vi "Valve_EPICS_Dev4_APX - Copy.vi"() -> ()   [LabVIEW 2015]
uses:
  <vilib>/Platform/TimedLoop/XDataNode/timing_clust.ctl
  <vilib>/Platform/TimedLoop/XDataNode/nitl_modes.ctl
  <vilib>/Platform/TimedLoop/XDataNode/wakeup.ctl
  <userlib>/caLab/Private/Get_PV-1D.vi
  <userlib>/caLab/Private/Put_DBL-1D_PV-1D.vi
  <vilib>/platform/TimedLoop/XDataNode/XDataNode.xnode
  <vilib>/Platform/TimedLoop/XDataNode/XDNodeRunTimeDep.lvlib
panel:
  out "Vacuum_REQ":bool
  out "Ambient_REQ":bool
  out "V7_CLOSE_REQ":bool
  out "V6_CLOSE_REQ":bool
  out "V5_CLOSE_REQ":bool
  out "V4_CLOSE_REQ":bool
  out "V3_CLOSE_REQ":bool
  out "V2_CLOSE_REQ":bool
  out "V1_CLOSE_REQ":bool
  out "V0_CLOSE_REQ":bool
  out "V7_OPEN_REQ":bool
  out "V6_OPEN_REQ":bool
  out "V5_OPEN_REQ":bool
  out "V4_OPEN_REQ":bool
  out "V3_OPEN_REQ":bool
  out "V2_OPEN_REQ":bool
  out "V1_OPEN_REQ":bool
  out "V0_OPEN_REQ":bool
  out "V7_OPEN_ENB":bool
  out "V6_OPEN_ENB":bool
  out "V5_OPEN_ENB":bool
  out "V4_OPEN_ENB":bool
  out "V3_OPEN_ENB":bool
  out "V2_OPEN_ENB":bool
  out "V1_OPEN_ENB":bool
  out "V0_OPEN_ENB":bool
  out "Boolean array":bool[](array[boolean])
  out "V7_OPEN_ACT":bool
  out "V6_OPEN_ACT":bool
  out "V5_OPEN_ACT":bool
  out "V4_OPEN_ACT":bool
  out "V3_OPEN_ACT":bool
  out "V2_OPEN_ACT":bool
  out "V1_OPEN_ACT":bool
  out "V0_OPEN_ACT":bool
  out "initialized array":i16[](array[numeric])
  in  "stop":bool
  out "sum":i16
  out "0, 1":i16[](array[numeric])
  out "SCL_data":u32[](array[numeric]) caption="SCL"
  out "SOP_data":u32[](array[numeric]) caption="SOP"
  out "SCL7":bool
  out "SCL6":bool
  out "SCL5":bool
  out "SCL4":bool
  out "SCL3":bool
  out "SCL2":bool
  out "SCL1":bool
  out "SCL0":bool
  out "SOP7":bool
  out "SOP6":bool
  out "SOP5":bool
  out "SOP4":bool
  out "SOP3":bool
  out "SOP2":bool
  out "SOP1":bool
  out "SOP0":bool
  # "Valve control DEV4"
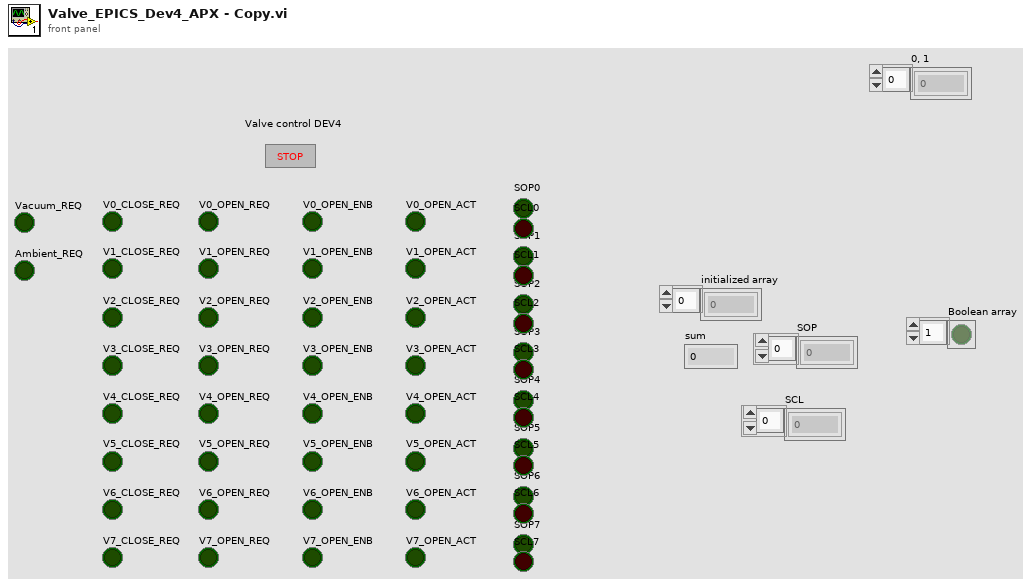
[diagram p1: front panel]
types:
  T1 = typedef "XDNodeRunTimeDep.lvlib/timing_clust.ctl" = cluster{"Expected End [f-1]":u64, "Actual End [f-1]":u64, "Finished Late? [f-1]":bool, "Expected End [i-1]":u64, "Actual End [i-1]":u64, "Finished Late? [i-1]":bool, "Expected Start [i]":u64, "Actual Start [i]":u64, "Expected Start [f]":u64, "Actual Start [f]":u64, "Source Name":string, "Structure Name":string, "Period":i64, "Deadline":i64, "Offset":i64, "Start":i64, "Priority":i32, "Timeout":i32, "Mode":T2, "Wakeup Reason":T3, "Error":errorcluster, "Source Type":string, "Secondary Source Type":string, "Global End Time":u64, "Global Start Time":u64, "Frame Duration":u64, "Iteration Duration":u64, "Assigned CPU":i32, "I/O Scan Engine Mode":u32}
  T2 = typedef "XDNodeRunTimeDep.lvlib/nitl_modes.ctl" = enum32{"No Change", "Process missed periods, maintain original phase", "Discard missed periods, maintain original phase", "Process missed periods, ignore original phase", "Discard missed periods, ignore original phase"}
  T3 = typedef "XDNodeRunTimeDep.lvlib/wakeup.ctl" = enum32{"Normal", "Aborted", "Asynchronous wakeup", "Timing source error", "Timed loop error", "Timeout"}
  T4 = typedef "NI_Matrix.lvlib/RealMatrix.ctl" = dbl[][]
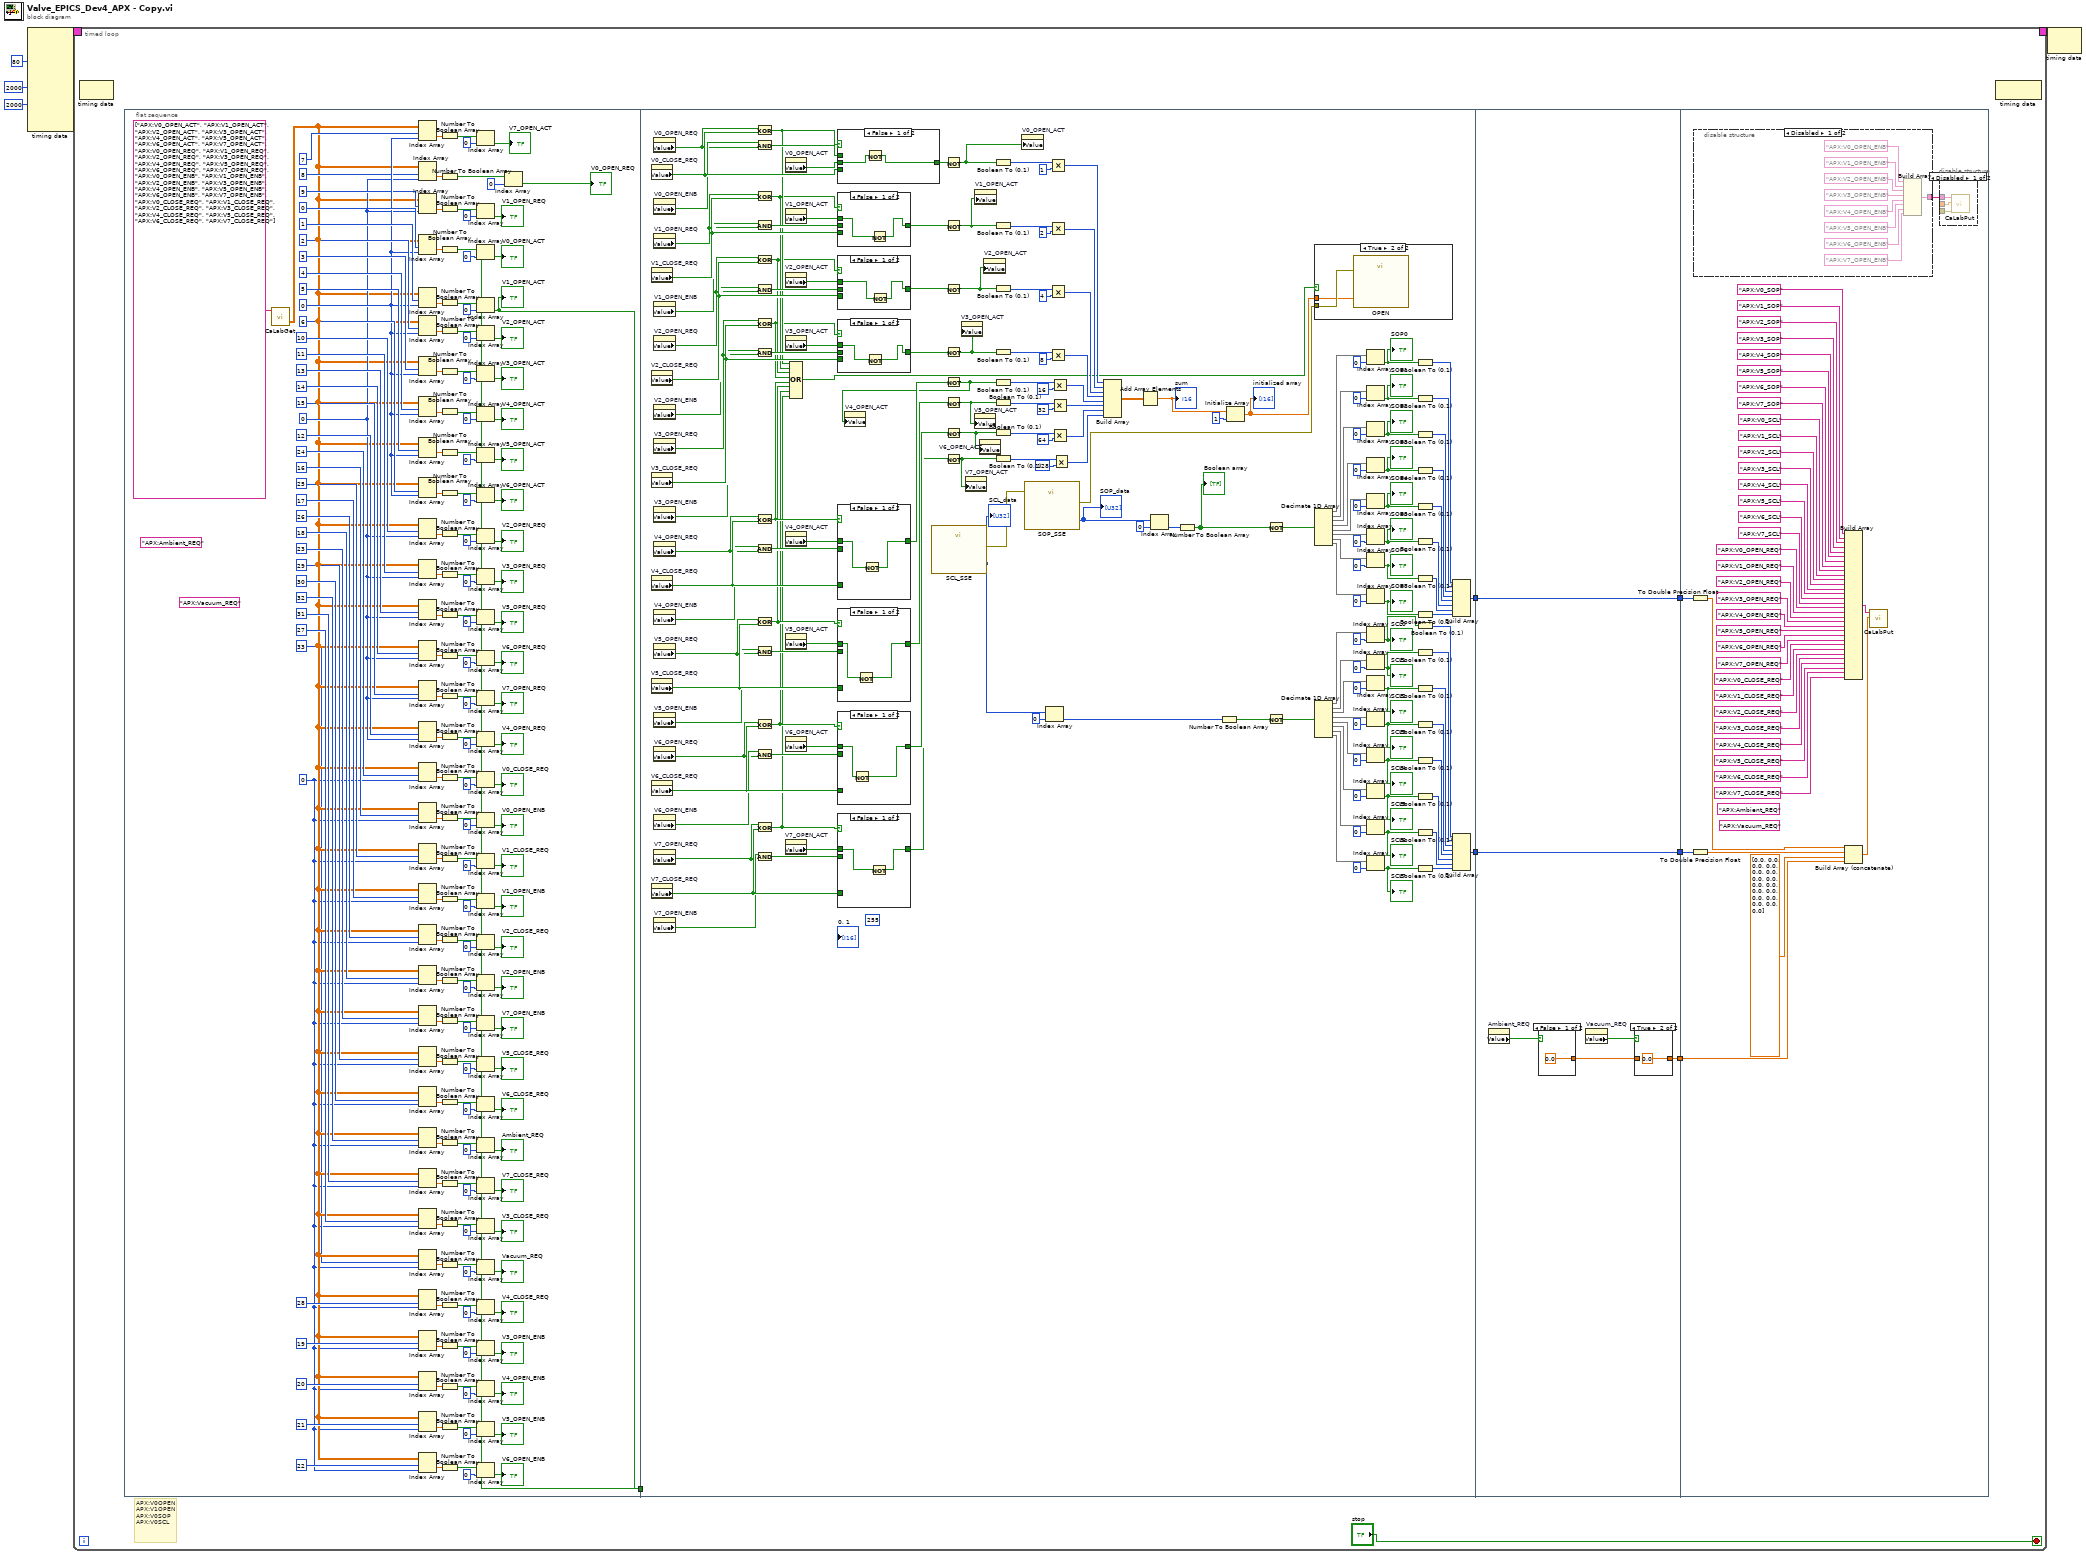
[diagram p0: block diagram]
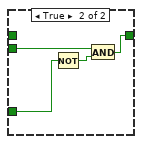
[diagram p3: hidden frame]
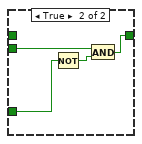
[diagram p4: hidden frame]
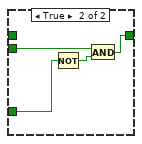
[diagram p5: hidden frame]
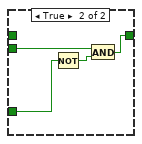
[diagram p6: hidden frame]
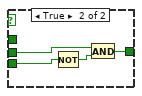
[diagram p7: hidden frame]
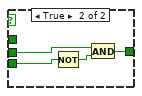
[diagram p8: hidden frame]
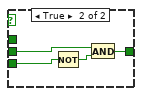
[diagram p9: hidden frame]
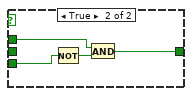
[diagram p10: hidden frame]
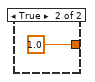
[diagram p12: hidden frame]
diagram:
  n1 = node-c288(80 ("Priority"), i64 2000 ("Deadline"), 2000 ("Timeout")) -> (w5:T1)  [unwired: 7 in]
  n2 = timed-loop {
    timing: w5 -> [_]
    timing-out: [_] -> w4
    stop <- "stop" stop-if-true
    # "APX:V0OPEN\nAPX:V1OPEN\nAPX:V0SOP\nAPX:V0SCL"
    n3 = node-c288() -> ()  [unwired: 1 in, 1 out]
    n4 = flat-sequence {
      tunnel: [w78] -> w18
      tunnel: [w77] -> w17
      tunnel: [w73] -> w16
      tunnel: [w80] -> w15
      tunnel: [w79] -> w14
      tunnel: [w76] -> w13
      tunnel: [w75] -> w12
      tunnel: w18 -> [_]
      tunnel: w17 -> [_]
      tunnel: w16 -> [_]
      tunnel: w15 -> [_]
      tunnel: w14 -> [_]
      tunnel: w13 -> [_]
      tunnel: w12 -> [_]
      tunnel: [w270] -> w11
      tunnel: [w343] -> w8
      tunnel: w11 -> [w422]
      tunnel: [w422] -> w10
      tunnel: w8 -> [w421]
      tunnel: [w421] -> w7
      tunnel: [w417] -> w6
      tunnel: w10 -> [w467]
      tunnel: w7 -> [w466]
      tunnel: w6 -> [w427]
      frame #0 {
        (unwired) "APX:Vacuum_REQ"
        (unwired) "APX:Ambient_REQ"
        w24 = 0 ("index")
        w153 = 0 ("index")
        w186 = 0 ("index")
        n5 = call-poly "CaLabGet.vi"("PV Names"=string[] ["APX:V0_OPEN_ACT", "APX:V1_OPEN_ACT", "APX:V2_OPEN_ACT", "APX:V3_OPEN_ACT", "APX:V4_OPEN_ACT", "APX:V5_OPEN_ACT", "APX:V6_OPEN_ACT", "APX:V7_OPEN_ACT", "APX:V0_OPEN_REQ", "APX:V1_OPEN_REQ", "APX:V2_OPEN_REQ", "APX:V3_OPEN_REQ", "APX:V4_OPEN_REQ", "APX:V5_OPEN_REQ", "APX:V6_OPEN_REQ", "APX:V7_OPEN_REQ", "APX:V0_OPEN_ENB", "APX:V1_OPEN_ENB", "APX:V2_OPEN_ENB", "APX:V3_OPEN_ENB", "APX:V4_OPEN_ENB", "APX:V5_OPEN_ENB", "APX:V6_OPEN_ENB", "APX:V7_OPEN_ENB", "APX:V0_CLOSE_REQ", "APX:V1_CLOSE_REQ", "APX:V2_CLOSE_REQ", "APX:V3_CLOSE_REQ", "APX:V4_CLOSE_REQ", "APX:V5_CLOSE_REQ", "APX:V6_CLOSE_REQ", "APX:V7_CLOSE_REQ"]) -> ("Value Array (number)"=w26:dbl[][])  [unwired: 8 in, 6 out]
        n6 = Index Array(array=w26, index (row)=7, index (col)=w186) -> (element=w162:dbl)
        n7 = Index Array(array=w26, index (row)=8 ("disabled index (row)"), index (col)=w153) -> (element=w133:dbl)
        n8 = Index Array(array=w26, index (row)=9, index (col)=w153) -> (element=w132:dbl)
        n9 = Index Array(array=w26, index (row)=0 ("disabled index (row)"), index (col)=w186) -> (element=w166:dbl)
        n10 = Index Array(array=w26, index (row)=1, index (col)=w186) -> (element=w165:dbl)
        n11 = Index Array(array=w26, index (row)=2, index (col)=w186) -> (element=w169:dbl)
        n12 = Index Array(array=w26, index (row)=3 ("index"), index (col)=w186) -> (element=w168:dbl)
        n13 = Index Array(array=w26, index (row)=4, index (col)=w186) -> (element=w167:dbl)
        n14 = Index Array(array=w26, index (row)=5, index (col)=w186) -> (element=w164:dbl)
        n15 = Index Array(array=w26, index (row)=6, index (col)=w186) -> (element=w163:dbl)
        n16 = Index Array(array=w26, index (row)=10, index (col)=w153) -> (element=w136:dbl)
        n17 = Index Array(array=w26, index (row)=11 ("index"), index (col)=w153) -> (element=w135:dbl)
        n18 = Index Array(array=w26, index (row)=13, index (col)=w153) -> (element=w131:dbl)
        n19 = Index Array(array=w26, index (row)=14, index (col)=w153) -> (element=w130:dbl)
        n20 = Index Array(array=w26, index (row)=15, index (col)=w153) -> (element=w129:dbl)
        n21 = Index Array(array=w26, index (row)=12, index (col)=w153) -> (element=w134:dbl)
        n22 = Index Array(array=w26, index (row)=24, index (col)=w24) -> (element=w53:dbl)
        n23 = Index Array(array=w26, index (row)=16 ("disabled index (row)"), index (col)=w24) -> (element=w101:dbl)
        n24 = Index Array(array=w26, index (row)=25, index (col)=w24) -> (element=w52:dbl)
        n25 = Index Array(array=w26, index (row)=17, index (col)=w24) -> (element=w100:dbl)
        n26 = Index Array(array=w26, index (row)=26, index (col)=w24) -> (element=w56:dbl)
        n27 = Index Array(array=w26, index (row)=18, index (col)=w24) -> (element=w104:dbl)
        n28 = Index Array(array=w26, index (row)=23, index (col)=w24) -> (element=w97:dbl)
        n29 = Index Array(array=w26, index (row)=29, index (col)=w24) -> (element=w51:dbl)
        n30 = Index Array(array=w26, index (row)=30, index (col)=w24) -> (element=w50:dbl)
        n31 = Index Array(array=w26, index (row)=32, index (col)=w24) -> (element=w30:dbl)
        n32 = Index Array(array=w26, index (row)=31, index (col)=w24) -> (element=w49:dbl)
        n33 = Index Array(array=w26, index (row)=27, index (col)=w24) -> (element=w55:dbl)
        n34 = Index Array(array=w26, index (row)=33, index (col)=w24) -> (element=w27:dbl)
        n35 = Index Array(array=w26, index (row)=28, index (col)=w24) -> (element=w54:dbl)
        n36 = Index Array(array=w26, index (row)=19 ("index"), index (col)=w24) -> (element=w103:dbl)
        n37 = Index Array(array=w26, index (row)=20, index (col)=w24) -> (element=w102:dbl)
        n38 = Index Array(array=w26, index (row)=21, index (col)=w24) -> (element=w99:dbl)
        n39 = Index Array(array=w26, index (row)=22, index (col)=w24) -> (element=w98:dbl)
        n40 = Number To Boolean Array(number=w162) -> (Boolean array=w171:bool[])
        n41 = Number To Boolean Array(number=w133) -> (Boolean array=w146:bool[])
        n42 = Number To Boolean Array(number=w132) -> (Boolean array=w144:bool[])
        n43 = Number To Boolean Array(number=w166) -> (Boolean array=w179:bool[])
        n44 = Number To Boolean Array(number=w165) -> (Boolean array=w177:bool[])
        n45 = Number To Boolean Array(number=w169) -> (Boolean array=w185:bool[])
        n46 = Number To Boolean Array(number=w168) -> (Boolean array=w183:bool[])
        n47 = Number To Boolean Array(number=w167) -> (Boolean array=w181:bool[])
        n48 = Number To Boolean Array(number=w164) -> (Boolean array=w175:bool[])
        n49 = Number To Boolean Array(number=w163) -> (Boolean array=w173:bool[])
        n50 = Number To Boolean Array(number=w136) -> (Boolean array=w152:bool[])
        n51 = Number To Boolean Array(number=w135) -> (Boolean array=w150:bool[])
        n52 = Number To Boolean Array(number=w131) -> (Boolean array=w142:bool[])
        n53 = Number To Boolean Array(number=w130) -> (Boolean array=w140:bool[])
        n54 = Number To Boolean Array(number=w129) -> (Boolean array=w138:bool[])
        n55 = Number To Boolean Array(number=w134) -> (Boolean array=w148:bool[])
        n56 = Number To Boolean Array(number=w53) -> (Boolean array=w66:bool[])
        n57 = Number To Boolean Array(number=w101) -> (Boolean array=w114:bool[])
        n58 = Number To Boolean Array(number=w52) -> (Boolean array=w64:bool[])
        n59 = Number To Boolean Array(number=w100) -> (Boolean array=w112:bool[])
        n60 = Number To Boolean Array(number=w56) -> (Boolean array=w72:bool[])
        n61 = Number To Boolean Array(number=w104) -> (Boolean array=w120:bool[])
        n62 = Number To Boolean Array(number=w97) -> (Boolean array=w106:bool[])
        n63 = Number To Boolean Array(number=w51) -> (Boolean array=w62:bool[])
        n64 = Number To Boolean Array(number=w50) -> (Boolean array=w60:bool[])
        n65 = Number To Boolean Array(number=w30) -> (Boolean array=w32:bool[])
        n66 = Number To Boolean Array(number=w49) -> (Boolean array=w58:bool[])
        n67 = Number To Boolean Array(number=w55) -> (Boolean array=w70:bool[])
        n68 = Number To Boolean Array(number=w27) -> (Boolean array=w23:bool[])
        n69 = Number To Boolean Array(number=w54) -> (Boolean array=w68:bool[])
        n70 = Number To Boolean Array(number=w103) -> (Boolean array=w118:bool[])
        n71 = Number To Boolean Array(number=w102) -> (Boolean array=w116:bool[])
        n72 = Number To Boolean Array(number=w99) -> (Boolean array=w110:bool[])
        n73 = Number To Boolean Array(number=w98) -> (Boolean array=w108:bool[])
        n74 = Index Array(array=w171, index=0) -> (element=→"V7_OPEN_ACT":bool)
        n75 = Index Array(array=w144, index=0) -> (element=→"V1_OPEN_REQ":bool)
        n76 = Index Array(array=w179, index=0) -> (element=w80:bool)
        "V0_OPEN_ACT" <- w80
        n77 = Index Array(array=w177, index=0) -> (element=w79:bool)
        "V1_OPEN_ACT" <- w79
        n78 = Index Array(array=w185, index=0) -> (element=w78:bool)
        "V2_OPEN_ACT" <- w78
        n79 = Index Array(array=w183, index=0) -> (element=w77:bool)
        "V3_OPEN_ACT" <- w77
        n80 = Index Array(array=w181, index=0) -> (element=w73:bool)
        "V4_OPEN_ACT" <- w73
        n81 = Index Array(array=w175, index=0) -> (element=w76:bool)
        "V5_OPEN_ACT" <- w76
        n82 = Index Array(array=w173, index=0) -> (element=w75:bool)
        "V6_OPEN_ACT" <- w75
        n83 = Index Array(array=w152, index=0) -> (element=→"V2_OPEN_REQ":bool)
        n84 = Index Array(array=w150, index=0) -> (element=→"V3_OPEN_REQ":bool)
        n85 = Index Array(array=w142, index=0) -> (element=→"V5_OPEN_REQ":bool)
        n86 = Index Array(array=w140, index=0) -> (element=→"V6_OPEN_REQ":bool)
        n87 = Index Array(array=w138, index=0) -> (element=→"V7_OPEN_REQ":bool)
        n88 = Index Array(array=w148, index=0) -> (element=→"V4_OPEN_REQ":bool)
        n89 = Index Array(array=w66, index=0) -> (element=→"V0_CLOSE_REQ":bool)
        n90 = Index Array(array=w114, index=0) -> (element=→"V0_OPEN_ENB":bool)
        n91 = Index Array(array=w64, index=0) -> (element=→"V1_CLOSE_REQ":bool)
        n92 = Index Array(array=w112, index=0) -> (element=→"V1_OPEN_ENB":bool)
        n93 = Index Array(array=w72, index=0) -> (element=→"V2_CLOSE_REQ":bool)
        n94 = Index Array(array=w120, index=0) -> (element=→"V2_OPEN_ENB":bool)
        n95 = Index Array(array=w106, index=0) -> (element=→"V7_OPEN_ENB":bool)
        n96 = Index Array(array=w62, index=0) -> (element=→"V5_CLOSE_REQ":bool)
        n97 = Index Array(array=w60, index=0) -> (element=→"V6_CLOSE_REQ":bool)
        n98 = Index Array(array=w32, index=0) -> (element=→"Ambient_REQ":bool)
        n99 = Index Array(array=w58, index=0) -> (element=→"V7_CLOSE_REQ":bool)
        n100 = Index Array(array=w70, index=0) -> (element=→"V3_CLOSE_REQ":bool)
        n101 = Index Array(array=w23, index=0) -> (element=→"Vacuum_REQ":bool)
        n102 = Index Array(array=w68, index=0) -> (element=→"V4_CLOSE_REQ":bool)
        n103 = Index Array(array=w118, index=0) -> (element=→"V3_OPEN_ENB":bool)
        n104 = Index Array(array=w116, index=0) -> (element=→"V4_OPEN_ENB":bool)
        n105 = Index Array(array=w110, index=0) -> (element=→"V5_OPEN_ENB":bool)
        n106 = Index Array(array=w108, index=0) -> (element=→"V6_OPEN_ENB":bool)
        n107 = Index Array "Index Array"(array=w146, index=0) -> (element=→"V0_OPEN_REQ":bool)
      }
      frame #1 {
        (unwired) u32 255 ("y")
        n108 = property on="V0_CLOSE_REQ" class="Bool (strict)"() -> ("Value"=w260:bool)  [unwired: 2 in, 2 out]
        n109 = property on="V1_CLOSE_REQ" class="Bool (strict)"() -> ("Value"=w255:bool)  [unwired: 2 in, 2 out]
        n110 = property on="V2_CLOSE_REQ" class="Bool (strict)"() -> ("Value"=w250:bool)  [unwired: 2 in, 2 out]
        n111 = property on="V3_CLOSE_REQ" class="Bool (strict)"() -> ("Value"=w245:bool)  [unwired: 2 in, 2 out]
        n112 = property on="V4_CLOSE_REQ" class="Bool (strict)"() -> ("Value"=w240:bool)  [unwired: 2 in, 2 out]
        n113 = property on="V5_CLOSE_REQ" class="Bool (strict)"() -> ("Value"=w235:bool)  [unwired: 2 in, 2 out]
        n114 = property on="V6_CLOSE_REQ" class="Bool (strict)"() -> ("Value"=w230:bool)  [unwired: 2 in, 2 out]
        n115 = property on="V7_CLOSE_REQ" class="Bool (strict)"() -> ("Value"=w225:bool)  [unwired: 2 in, 2 out]
        n116 = property on="V0_OPEN_REQ" class="Bool (strict)"() -> ("Value"=w258:bool)  [unwired: 2 in, 2 out]
        n117 = property on="V0_OPEN_ENB" class="Bool (strict)"() -> ("Value"=w259:bool)  [unwired: 2 in, 2 out]
        n118 = property on="V1_OPEN_REQ" class="Bool (strict)"() -> ("Value"=w253:bool)  [unwired: 2 in, 2 out]
        n119 = property on="V1_OPEN_ENB" class="Bool (strict)"() -> ("Value"=w254:bool)  [unwired: 2 in, 2 out]
        n120 = property on="V2_OPEN_REQ" class="Bool (strict)"() -> ("Value"=w248:bool)  [unwired: 2 in, 2 out]
        n121 = property on="V2_OPEN_ENB" class="Bool (strict)"() -> ("Value"=w249:bool)  [unwired: 2 in, 2 out]
        n122 = property on="V3_OPEN_REQ" class="Bool (strict)"() -> ("Value"=w243:bool)  [unwired: 2 in, 2 out]
        n123 = property on="V3_OPEN_ENB" class="Bool (strict)"() -> ("Value"=w244:bool)  [unwired: 2 in, 2 out]
        n124 = property on="V4_OPEN_REQ" class="Bool (strict)"() -> ("Value"=w238:bool)  [unwired: 2 in, 2 out]
        n125 = property on="V4_OPEN_ENB" class="Bool (strict)"() -> ("Value"=w239:bool)  [unwired: 2 in, 2 out]
        n126 = property on="V5_OPEN_REQ" class="Bool (strict)"() -> ("Value"=w233:bool)  [unwired: 2 in, 2 out]
        n127 = property on="V5_OPEN_ENB" class="Bool (strict)"() -> ("Value"=w234:bool)  [unwired: 2 in, 2 out]
        n128 = property on="V6_OPEN_REQ" class="Bool (strict)"() -> ("Value"=w228:bool)  [unwired: 2 in, 2 out]
        n129 = property on="V6_OPEN_ENB" class="Bool (strict)"() -> ("Value"=w229:bool)  [unwired: 2 in, 2 out]
        n130 = property on="V7_OPEN_REQ" class="Bool (strict)"() -> ("Value"=w223:bool)  [unwired: 2 in, 2 out]
        n131 = property on="V7_OPEN_ENB" class="Bool (strict)"() -> ("Value"=w224:bool)  [unwired: 2 in, 2 out]
        n132 = Exclusive Or(1:w260, 2:w258) -> (0:w219:bool)
        n133 = And(x=w259, y=w258) -> (x .and. y?=w257:bool)
        n134 = Exclusive Or(1:w255, 2:w253) -> (0:w218:bool)
        n135 = And(x=w254, y=w253) -> (x .and. y?=w252:bool)
        n136 = Exclusive Or(1:w250, 2:w248) -> (0:w217:bool)
        n137 = And(x=w249, y=w248) -> (x .and. y?=w247:bool)
        n138 = Exclusive Or(1:w245, 2:w243) -> (0:w216:bool)
        n139 = And(x=w244, y=w243) -> (x .and. y?=w242:bool)
        n140 = Exclusive Or(1:w240, 2:w238) -> (0:w215:bool)
        n141 = And(x=w239, y=w238) -> (x .and. y?=w237:bool)
        n142 = Exclusive Or(1:w235, 2:w233) -> (0:w214:bool)
        n143 = And(x=w234, y=w233) -> (x .and. y?=w232:bool)
        n144 = Exclusive Or(1:w230, 2:w228) -> (0:w213:bool)
        n145 = And(x=w229, y=w228) -> (x .and. y?=w227:bool)
        n146 = Exclusive Or(1:w225, 2:w223) -> (0:w212:bool)
        n147 = And(x=w224, y=w223) -> (x .and. y?=w222:bool)
        n148 = property on="V0_OPEN_ACT" class="Bool (strict)"() -> ("Value"=w256:bool)  [unwired: 2 in, 2 out]
        n149 = property on="V1_OPEN_ACT" class="Bool (strict)"() -> ("Value"=w251:bool)  [unwired: 2 in, 2 out]
        n150 = property on="V2_OPEN_ACT" class="Bool (strict)"() -> ("Value"=w246:bool)  [unwired: 2 in, 2 out]
        n151 = property on="V3_OPEN_ACT" class="Bool (strict)"() -> ("Value"=w241:bool)  [unwired: 2 in, 2 out]
        n152 = property on="V4_OPEN_ACT" class="Bool (strict)"() -> ("Value"=w236:bool)  [unwired: 2 in, 2 out]
        n153 = property on="V5_OPEN_ACT" class="Bool (strict)"() -> ("Value"=w231:bool)  [unwired: 2 in, 2 out]
        n154 = property on="V6_OPEN_ACT" class="Bool (strict)"() -> ("Value"=w226:bool)  [unwired: 2 in, 2 out]
        n155 = property on="V7_OPEN_ACT" class="Bool (strict)"() -> ("Value"=w221:bool)  [unwired: 2 in, 2 out]
        n156 = Compound Arithmetic op=OR(w219, w218, w217, w216, w215, w214, w213, w212) -> (w220:bool)
        n157 = case shown="False" w219 {
          tunnel: w260 -> [_ w416]
          tunnel: w257 -> [_ w415]
          tunnel: [w411 w413] -> w211
          tunnel: w256 -> [w412 _]
          frame False {
            n158 = Not(x=w412) -> (.not. x?=w411:bool)
          }
          frame True {
            n159 = Not(x=w416) -> (.not. x?=w414:bool)
            n160 = And(x=w415, y=w414) -> (x .and. y?=w413:bool)
          }
        }
        n161 = case shown="False" w218 {
          tunnel: w255 -> [_ w410]
          tunnel: w252 -> [_ w409]
          tunnel: [w405 w407] -> w210
          tunnel: w251 -> [w406 _]
          frame False {
            n162 = Not(x=w406) -> (.not. x?=w405:bool)
          }
          frame True {
            n163 = Not(x=w410) -> (.not. x?=w408:bool)
            n164 = And(x=w409, y=w408) -> (x .and. y?=w407:bool)
          }
        }
        n165 = case shown="False" w217 {
          tunnel: w250 -> [_ w404]
          tunnel: w247 -> [_ w403]
          tunnel: [w399 w401] -> w209
          tunnel: w246 -> [w400 _]
          frame False {
            n166 = Not(x=w400) -> (.not. x?=w399:bool)
          }
          frame True {
            n167 = Not(x=w404) -> (.not. x?=w402:bool)
            n168 = And(x=w403, y=w402) -> (x .and. y?=w401:bool)
          }
        }
        n169 = case shown="False" w216 {
          tunnel: w245 -> [_ w398]
          tunnel: w242 -> [_ w397]
          tunnel: [w393 w395] -> w208
          tunnel: w241 -> [w394 _]
          frame False {
            n170 = Not(x=w394) -> (.not. x?=w393:bool)
          }
          frame True {
            n171 = Not(x=w398) -> (.not. x?=w396:bool)
            n172 = And(x=w397, y=w396) -> (x .and. y?=w395:bool)
          }
        }
        n173 = case shown="False" w215 {
          tunnel: w240 -> [_ w392]
          tunnel: w237 -> [_ w391]
          tunnel: [w387 w389] -> w207
          tunnel: w236 -> [w388 _]
          frame False {
            n174 = Not(x=w388) -> (.not. x?=w387:bool)
          }
          frame True {
            n175 = Not(x=w392) -> (.not. x?=w390:bool)
            n176 = And(x=w391, y=w390) -> (x .and. y?=w389:bool)
          }
        }
        n177 = case shown="False" w214 {
          tunnel: w235 -> [_ w386]
          tunnel: w232 -> [_ w385]
          tunnel: [w381 w383] -> w206
          tunnel: w231 -> [w382 _]
          frame False {
            n178 = Not(x=w382) -> (.not. x?=w381:bool)
          }
          frame True {
            n179 = Not(x=w386) -> (.not. x?=w384:bool)
            n180 = And(x=w385, y=w384) -> (x .and. y?=w383:bool)
          }
        }
        n181 = case shown="False" w213 {
          tunnel: w230 -> [_ w380]
          tunnel: w227 -> [_ w379]
          tunnel: [w375 w377] -> w205
          tunnel: w226 -> [w376 _]
          frame False {
            n182 = Not(x=w376) -> (.not. x?=w375:bool)
          }
          frame True {
            n183 = Not(x=w380) -> (.not. x?=w378:bool)
            n184 = And(x=w379, y=w378) -> (x .and. y?=w377:bool)
          }
        }
        n185 = case shown="False" w212 {
          tunnel: w225 -> [_ w374]
          tunnel: w222 -> [_ w373]
          tunnel: [w369 w371] -> w204
          tunnel: w221 -> [w370 _]
          frame False {
            n186 = Not(x=w370) -> (.not. x?=w369:bool)
          }
          frame True {
            n187 = Not(x=w374) -> (.not. x?=w372:bool)
            n188 = And(x=w373, y=w372) -> (x .and. y?=w371:bool)
          }
        }
        n189 = call "SCL_SSE"() -> ("data"=w298:u32[], "error out"=w357:errorcluster)  [unwired: 17 in, 1 out]
        "SCL_data" <- w298
        n190 = Not(x=w211) -> (.not. x?=w203:bool)
        n191 = Not(x=w210) -> (.not. x?=w202:bool)
        n192 = Not(x=w209) -> (.not. x?=w201:bool)
        n193 = Not(x=w208) -> (.not. x?=w200:bool)
        n194 = Not(x=w207) -> (.not. x?=w199:bool)
        n195 = property on="V4_OPEN_ACT" class="Bool (strict)"("Value"=w199) -> ()  [unwired: 2 in, 2 out]
        n196 = Not(x=w206) -> (.not. x?=w198:bool)
        n197 = Not(x=w205) -> (.not. x?=w197:bool)
        n198 = Not(x=w204) -> (.not. x?=w196:bool)
        n199 = property on="V3_OPEN_ACT" class="Bool (strict)"("Value"=w200) -> ()  [unwired: 2 in, 2 out]
        n200 = property on="V7_OPEN_ACT" class="Bool (strict)"("Value"=w196) -> ()  [unwired: 2 in, 2 out]
        n201 = property on="V5_OPEN_ACT" class="Bool (strict)"("Value"=w198) -> ()  [unwired: 2 in, 2 out]
        n202 = property on="V1_OPEN_ACT" class="Bool (strict)"("Value"=w202) -> ()  [unwired: 2 in, 2 out]
        n203 = property on="V6_OPEN_ACT" class="Bool (strict)"("Value"=w197) -> ()  [unwired: 2 in, 2 out]
        n204 = property on="V2_OPEN_ACT" class="Bool (strict)"("Value"=w201) -> ()  [unwired: 2 in, 2 out]
        n205 = Boolean To (0,1)(Boolean=w203) -> (0, 1=w342:i16)
        n206 = Boolean To (0,1)(Boolean=w202) -> (0, 1=w341:i16)
        n207 = Boolean To (0,1)(Boolean=w201) -> (0, 1=w340:i16)
        n208 = Boolean To (0,1)(Boolean=w200) -> (0, 1=w339:i16)
        n209 = Boolean To (0,1)(Boolean=w199) -> (0, 1=w338:i16)
        n210 = Boolean To (0,1)(Boolean=w198) -> (0, 1=w337:i16)
        n211 = Boolean To (0,1)(Boolean=w197) -> (0, 1=w336:i16)
        n212 = Boolean To (0,1)(Boolean=w196) -> (0, 1=w335:i16)
        n213 = property on="V0_OPEN_ACT" class="Bool (strict)"("Value"=w203) -> ()  [unwired: 2 in, 2 out]
        n214 = call "SOP_SSE"("error in"=w357) -> ("data"=w297:u32[], "error out"=w356:errorcluster)  [unwired: 16 in, 1 out]
        "SOP_data" <- w297
        n215 = Index Array(array=w298, index=0) -> (element=w316:u32)
        n216 = Multiply(x=w342, y=i16 1) -> (x*y=w326:i16)
        n217 = Multiply(x=w341, y=i16 2) -> (x*y=w325:i16)
        n218 = Multiply(x=w340, y=i16 4) -> (x*y=w324:i16)
        n219 = Multiply(x=w339, y=i16 8) -> (x*y=w323:i16)
        n220 = Multiply(x=w338, y=i16 16) -> (x*y=w322:i16)
        n221 = Multiply(x=w337, y=i16 32) -> (x*y=w321:i16)
        n222 = Multiply(x=w336, y=i16 64) -> (x*y=w320:i16)
        n223 = Multiply(x=w335, y=i16 128) -> (x*y=w319:i16)
        n224 = Build Array(w326, w325, w324, w323, w322, w321, w320, w319) -> (w318:T4)
        n225 = Add Array Elements(numeric array=w318) -> (sum=w354:dbl)
        "sum" <- w354
        n226 = Index Array(array=w297, index=0) -> (element=w317:u32)
        n227 = Number To Boolean Array(number=w317) -> (Boolean array=w296:bool[])
        "Boolean array" <- w296
        n228 = Number To Boolean Array(number=w316) -> (Boolean array=w307:bool[])
        n229 = Initialize Array(w354, 1 ("dimension size")) -> (w353:dbl[])
        "initialized array" <- w353
        n230 = Not(x=w296) -> (.not. x?=w295:bool[])
        n231 = Not(x=w307) -> (.not. x?=w294:bool[])
        n232 = case shown="True" w220 {
          tunnel: w356 -> [_ w368]
          tunnel: w353 -> [_ w367]
          frame False {
          }
          frame True {
            n233 = call "OPEN"("data"=w367, "error in"=w368) -> ()  [unwired: 16 in, 2 out]
          }
        }
        n234 = Decimate 1D Array(w295) -> (w315:bool[], w314:bool[], w313:bool[], w312:bool[], w311:bool[], w310:bool[], w309:bool[], w308:bool[])
        n235 = Decimate 1D Array(w294) -> (w306:bool[], w305:bool[], w304:bool[], w303:bool[], w302:bool[], w301:bool[], w300:bool[], w299:bool[])
        n236 = Index Array(array=w315, index=0) -> (element=w278:bool)
        "SOP0" <- w278
        n237 = Index Array(array=w314, index=0) -> (element=w293:bool)
        "SOP1" <- w293
        n238 = Index Array(array=w313, index=0) -> (element=w285:bool)
        "SOP2" <- w285
        n239 = Index Array(array=w312, index=0) -> (element=w284:bool)
        "SOP3" <- w284
        n240 = Index Array(array=w311, index=0) -> (element=w283:bool)
        "SOP4" <- w283
        n241 = Index Array(array=w310, index=0) -> (element=w282:bool)
        "SOP5" <- w282
        n242 = Index Array(array=w309, index=0) -> (element=w281:bool)
        "SOP6" <- w281
        n243 = Index Array(array=w308, index=0) -> (element=w280:bool)
        "SOP7" <- w280
        n244 = Index Array(array=w306, index=0) -> (element=w268:bool)
        "SCL0" <- w268
        n245 = Index Array(array=w305, index=0) -> (element=w267:bool)
        "SCL1" <- w267
        n246 = Index Array(array=w304, index=0) -> (element=w266:bool)
        "SCL2" <- w266
        n247 = Index Array(array=w303, index=0) -> (element=w265:bool)
        "SCL3" <- w265
        n248 = Index Array(array=w302, index=0) -> (element=w264:bool)
        "SCL4" <- w264
        n249 = Index Array(array=w301, index=0) -> (element=w263:bool)
        "SCL5" <- w263
        n250 = Index Array(array=w300, index=0) -> (element=w262:bool)
        "SCL6" <- w262
        n251 = Index Array(array=w299, index=0) -> (element=w261:bool)
        "SCL7" <- w261
        n252 = Boolean To (0,1)(Boolean=w278) -> (0, 1=w279:i16)
        n253 = Boolean To (0,1)(Boolean=w293) -> (0, 1=w292:i16)
        n254 = Boolean To (0,1)(Boolean=w285) -> (0, 1=w291:i16)
        n255 = Boolean To (0,1)(Boolean=w284) -> (0, 1=w290:i16)
        n256 = Boolean To (0,1)(Boolean=w283) -> (0, 1=w289:i16)
        n257 = Boolean To (0,1)(Boolean=w282) -> (0, 1=w288:i16)
        n258 = Boolean To (0,1)(Boolean=w281) -> (0, 1=w287:i16)
        n259 = Boolean To (0,1)(Boolean=w280) -> (0, 1=w286:i16)
        n260 = Boolean To (0,1)(Boolean=w268) -> (0, 1=w271:i16)
        n261 = Boolean To (0,1)(Boolean=w267) -> (0, 1=w277:i16)
        n262 = Boolean To (0,1)(Boolean=w266) -> (0, 1=w276:i16)
        n263 = Boolean To (0,1)(Boolean=w265) -> (0, 1=w275:i16)
        n264 = Boolean To (0,1)(Boolean=w264) -> (0, 1=w274:i16)
        n265 = Boolean To (0,1)(Boolean=w263) -> (0, 1=w273:i16)
        n266 = Boolean To (0,1)(Boolean=w262) -> (0, 1=w272:i16)
        n267 = Boolean To (0,1)(Boolean=w261) -> (0, 1=w269:i16)
        n268 = Build Array(w279, w292, w291, w290, w289, w288, w287, w286) -> (w343:i16[])
        n269 = Build Array(w271, w277, w276, w275, w274, w273, w272, w269) -> (w270:i16[])
      }
      frame #2 {
        n270 = property on="Ambient_REQ" class="Bool (strict)"() -> ("Value"=w420:bool)  [unwired: 2 in, 2 out]
        n271 = case shown="False" w420 {
          tunnel: [0.0 1.0] -> w418
          frame False {
          }
          frame True {
          }
        }
        n272 = property on="Vacuum_REQ" class="Bool (strict)"() -> ("Value"=w419:bool)  [unwired: 2 in, 2 out]
        n273 = case shown="True" w419 {
          tunnel: [w423 0.0] -> w417
          tunnel: w418 -> [w423 _]
          frame False {
          }
          frame True {
          }
        }
      }
      frame #3 {
        (unwired) "APX:Vacuum_REQ"
        (unwired) "APX:Ambient_REQ"
        n274 = To Double Precision Float(number=w466) -> (double precision float=w464:dbl[])
        n275 = To Double Precision Float(number=w467) -> (double precision float=w463:dbl[])
        n276 = disable-structure shown="Disabled" {
          disable-tunnel: [w471 _] -> w465
          frame Disabled {
            n277 = Build Array("APX:V0_OPEN_ENB", "APX:V1_OPEN_ENB", "APX:V2_OPEN_ENB", "APX:V3_OPEN_ENB", "APX:V4_OPEN_ENB", "APX:V5_OPEN_ENB", "APX:V6_OPEN_ENB", "APX:V7_OPEN_ENB") -> (w471:string[])
          }
          frame Enabled {
          }
        }
        n278 = Build Array("APX:V0_SOP", "APX:V1_SOP", "APX:V2_SOP", "APX:V3_SOP", "APX:V4_SOP", "APX:V5_SOP", "APX:V6_SOP", "APX:V7_SOP", "APX:V0_SCL", "APX:V1_SCL", "APX:V2_SCL", "APX:V3_SCL", "APX:V4_SCL", "APX:V5_SCL", "APX:V6_SCL", "APX:V7_SCL", "APX:V0_OPEN_REQ", "APX:V1_OPEN_REQ", "APX:V2_OPEN_REQ", "APX:V3_OPEN_REQ", "APX:V4_OPEN_REQ", "APX:V5_OPEN_REQ", "APX:V6_OPEN_REQ", "APX:V7_OPEN_REQ", "APX:V0_CLOSE_REQ", "APX:V1_CLOSE_REQ", "APX:V2_CLOSE_REQ", "APX:V3_CLOSE_REQ", "APX:V4_CLOSE_REQ", "APX:V5_CLOSE_REQ", "APX:V6_CLOSE_REQ", "APX:V7_CLOSE_REQ") -> (w429:string[])
        n279 = Build Array (concatenate)(w464, w463, dbl[] [0.0, 0.0, 0.0, 0.0, 0.0, 0.0, 0.0, 0.0, 0.0, 0.0, 0.0, 0.0, 0.0, 0.0, 0.0, 0.0, 0.0], w427) -> (w428:dbl[])
        n280 = call-poly <userlib>:"CaLabPut.vi"("Values"=w428, "PV Names"=w429) -> ()  [unwired: 6 in, 4 out]
        n281 = disable-structure shown="Disabled" {
          disable-tunnel: _ -> [w470 _]
          disable-tunnel: w465 -> [w469 _]
          disable-tunnel: _ -> [w468 _]
          frame Disabled {
            n282 = call-poly <userlib>:"CaLabPut.vi"("Error in (no error)"=w468, "Values"=w470, "PV Names"=w469) -> ()  [unwired: 5 in, 4 out]
          }
          frame Enabled {
          }
        }
      }
    }
    n283 = node-c288() -> ()  [unwired: 1 in, 1 out]
  }
  n284 = node-c288(w4) -> ()  [unwired: 1 out]
